vi "NXT_RestoreDefaultDisplay.vi"(11 "Sequence Flow in":T2) -> (3 "Sequence Flow out":T2)   [LabVIEW 2009]
doc: "Restores the NXT display to its default state."
uses:
  Library.llb/SequenceBoolean.ctl
  Library.llb/NXTSyscallRefnum.ctl
  C:/Program Files/National Instruments/LabVIEW 2009/resource/objmgr/NXTInputOutput.rc
panel:
  in  "Generic Refnum Name":T1
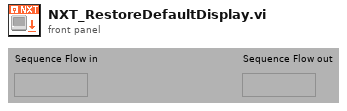
[diagram p1: front panel]
types:
  T1 = typedef "NXTSyscallRefnum.ctl" = refnum<k21>
  T2 = typedef "SequenceBoolean.ctl" = bool
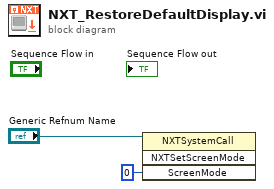
[diagram p0: block diagram]
diagram:
  n1 = invoke class="NXTSystemCall" method="NXTSetScreenMode"(reference="Generic Refnum Name", "ScreenMode"=u32 0) -> ()  [unwired: 2 in, 4 out]
